vi "Header_Info_Str.vi"(8 "error in (no error)":errorcluster, 11 "DefaultDev in":refnum<class "DefaultDev.lvclass">) -> (0 "error out":errorcluster, 1 "HdrInfoStr":string, 2 "InstrumentName":string, 3 "DefaultDev out":refnum<class "DefaultDev.lvclass">)   [LabVIEW 2012, in "DefaultDev.lvclass"]
uses:
  DefaultDev.lvclass
  DefaultDev.lvclass/DefaultDev.ctl
  DevicesClass/BaseDevice/BaseDevice.lvclass/BaseDevice.ctl
  DevicesClass/BaseDevice/Accessor/GetBeforewait(ms).vi
  DevicesClass/BaseDevice/Accessor/GetAfterwait(ms).vi
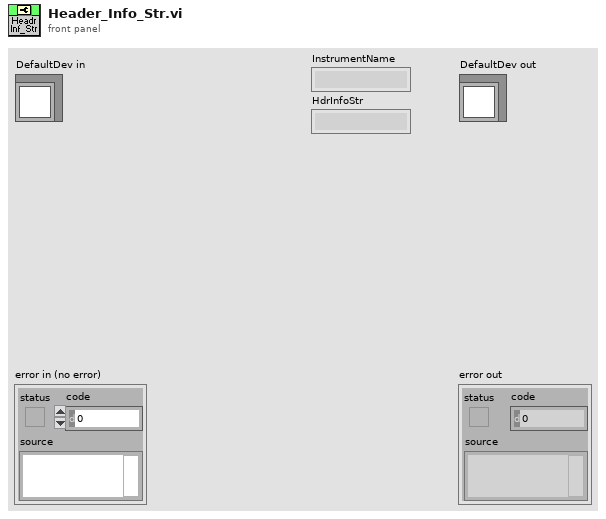
[diagram p1: front panel]
types:
  T1 = typedef "DefaultDev.lvclass/DefaultDev_Func.ctl" = enum16{"DefaultFunc (Arb)"}
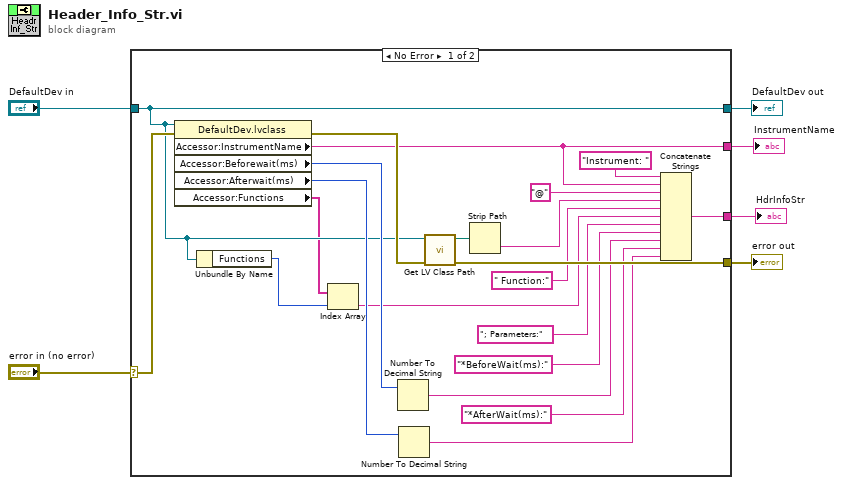
[diagram p0: block diagram]
diagram:
  n1 = case shown="No Error" "error in (no error)" {
    selector: "error in (no error)" -> [w23 w29]
    tunnel: [w21 w29] -> w5
    tunnel: [w13 w28] -> w3
    tunnel: "DefaultDev in" -> [w13 w28]
    tunnel: [w12 _] -> w2
    tunnel: [w7 _] -> w1
    frame No Error {
      n2 = property class="DefaultDev.lvclass"(reference=w13, error in=w23) -> (error out=w22:errorcluster, "Accessor:InstrumentName"=w12:string, "Accessor:Beforewait(ms)"=w20:u32, "Accessor:Afterwait(ms)"=w19:u32, "Accessor:Functions"=w11:string[])  [unwired: 1 out]
      n3 = Unbundle By Name(w13) -> ("Functions"=w10:T1)
      n4 = Index Array(array=w11, index=w10) -> (element=w9:string)
      n5 = Number To Decimal String(number=w20) -> (decimal integer string=w17:string)  [unwired: 1 in]
      n6 = Number To Decimal String(number=w19) -> (decimal integer string=w15:string)  [unwired: 1 in]
      n7 = call <vilib>:"Get LV Class Path.vi"("error in (no error)"=w22, "object"=w13) -> ("error out"=w21:errorcluster, "class path"=w24:path)  [unwired: 8 in]
      n8 = Strip Path(path=w24) -> (name=w26:string)  [unwired: 1 out]
      n9 = Concatenate Strings("Instrument: " ("string"), w12, "@" ("string"), w26, " Function:" ("Params"), w9, "; Parameters:" ("Params"), "*BeforeWait(ms):" ("Params"), w17, "*AfterWait(ms):" ("Params"), w15) -> (w7:string)
    }
    frame Error {
    }
  }
  "error out" <- w5
  "DefaultDev out" <- w3
  "InstrumentName" <- w2
  "HdrInfoStr" <- w1
